vi "SW_Load_settings_file_light.vi"   [LabVIEW 2016]
uses:
  <vilib>/Utility/config.llb/NI_LVConfig.lvlib
types:
  T1 = enum32{"invalid app kind", "Development System", "Run Time System", "Student Edition", "Embedded LabVIEW", "Evaluation", "Custom"}
  T2 = typedef "NI_LVConfig.lvlib/Config Data RefNum.ctl" = refnum<k1>
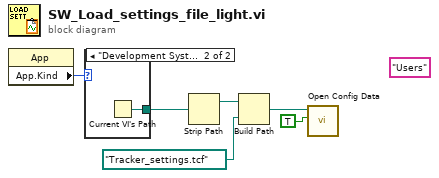
[diagram p0: block diagram]
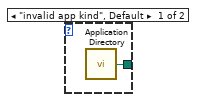
[diagram p2: hidden frame]
diagram:
  (unwired) "Users" ("Users section name")
  n1 = property class="App"() -> ("App.Kind"=w2:T1)  [unwired: 2 in, 2 out]
  n2 = case shown="\"Development System\"" w2 {
    tunnel: [w9 w10] -> w4
    frame "invalid app kind", Default {
      n3 = call <vilib>:"Application Directory.vi"() -> ("Application Directory"=w9:path)
    }
    frame "Development System" {
      n4 = Current VI's Path() -> (path=w10:path)
    }
  }
  n5 = Strip Path(path=w4) -> (stripped path=w5:path)  [unwired: 1 out]
  n6 = Build Path(base path=w5, name or relative path=path "Tracker_settings.tcf") -> (appended path=w1:path)
  n7 = call <vilib>:"Open Config Data.vi"("create file if necessary (T)"=TRUE, "configuration file path"=w1) -> ("error out"=w8:errorcluster, "refnum"=w7:T2)  [unwired: 7 in, 1 out]
